vi "Strategy 4_duty cycle variation_not working.vi"() -> ()   [LabVIEW 2018]
uses:
  <vilib>/DAQmx/write.llb/DAQmx Write (Digital 1D Bool 1Chan 1Samp).vi
  <vilib>/DAQmx/create/channels.llb/DAQmx Create Channel (DO-Digital Output).vi
  <vilib>/DAQmx/miscellaneous.llb/DAQmx Fill In Error Info.vi
  <vilib>/Waveform/DWDTOps.llb/DWDT Analog to Digital.vi
  <vilib>/Waveform/DWDTOps.llb/DWDT Digital to Boolean Array.vi
  <vilib>/ptbypt/NI_PtbyPt.lvlib
  <vilib>/measure/NI_MABase.lvlib
panel:
  out "Meter":dbl(knob) scale=0.0..100.0
  out "?":bool
  in  "Boolean":bool
  in  "sample length":i32=50
  out "Waveform Chart":dbl(graph)
  in  "Set Point":dbl(slide) scale=0.0..40.0
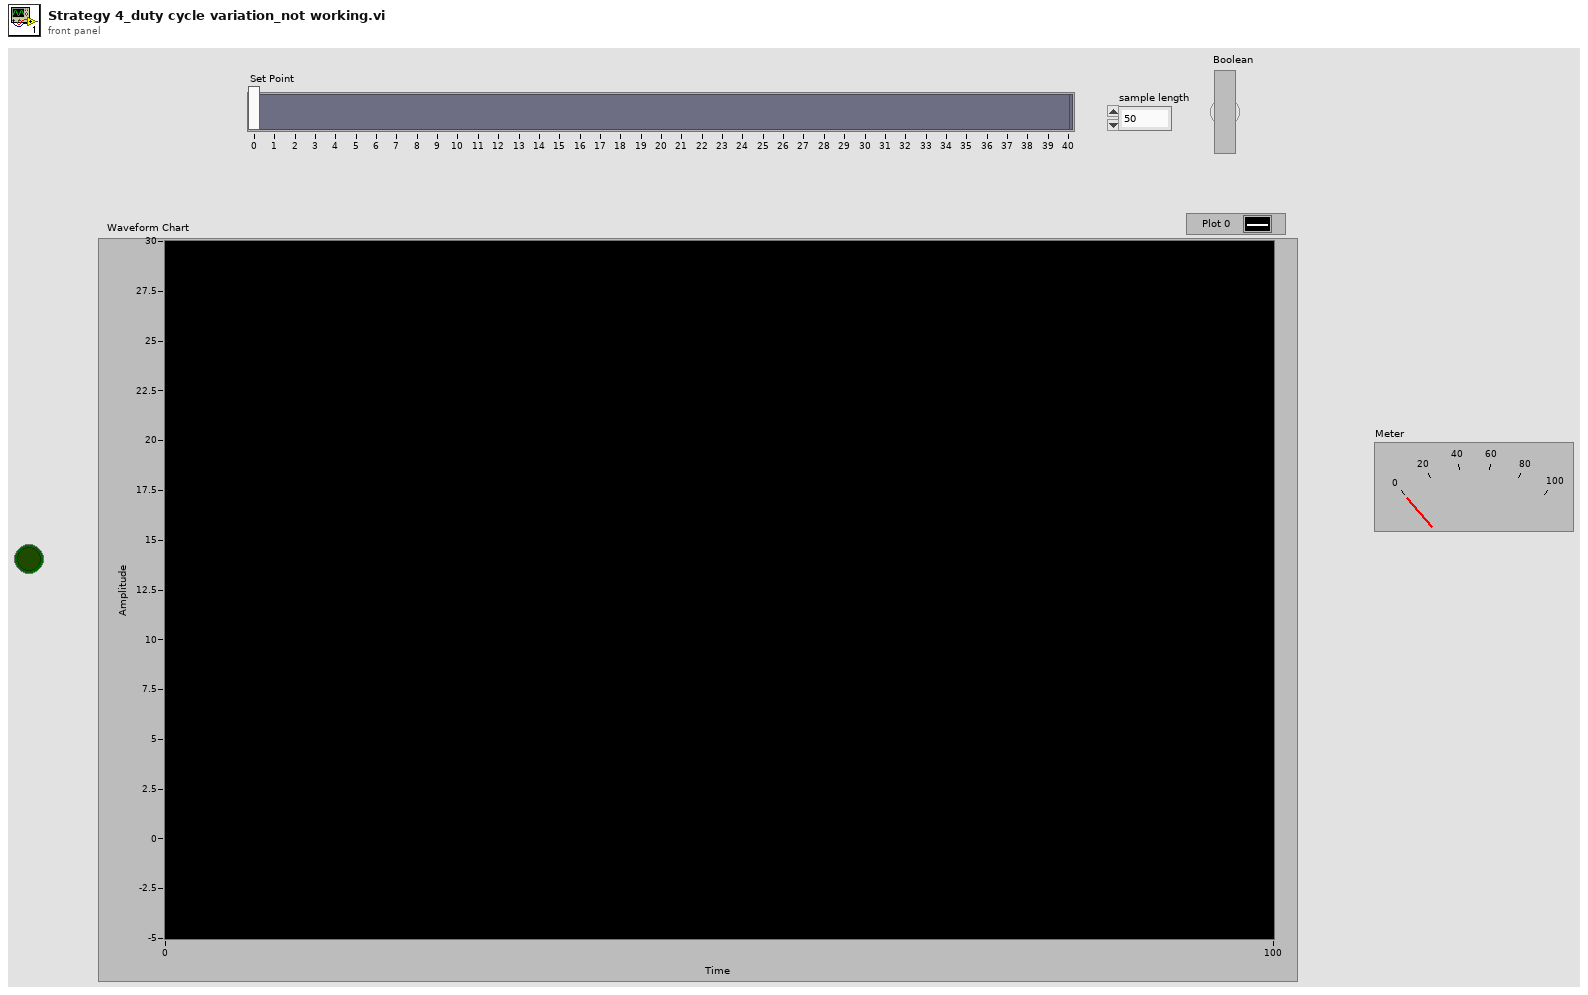
[diagram p1: front panel]
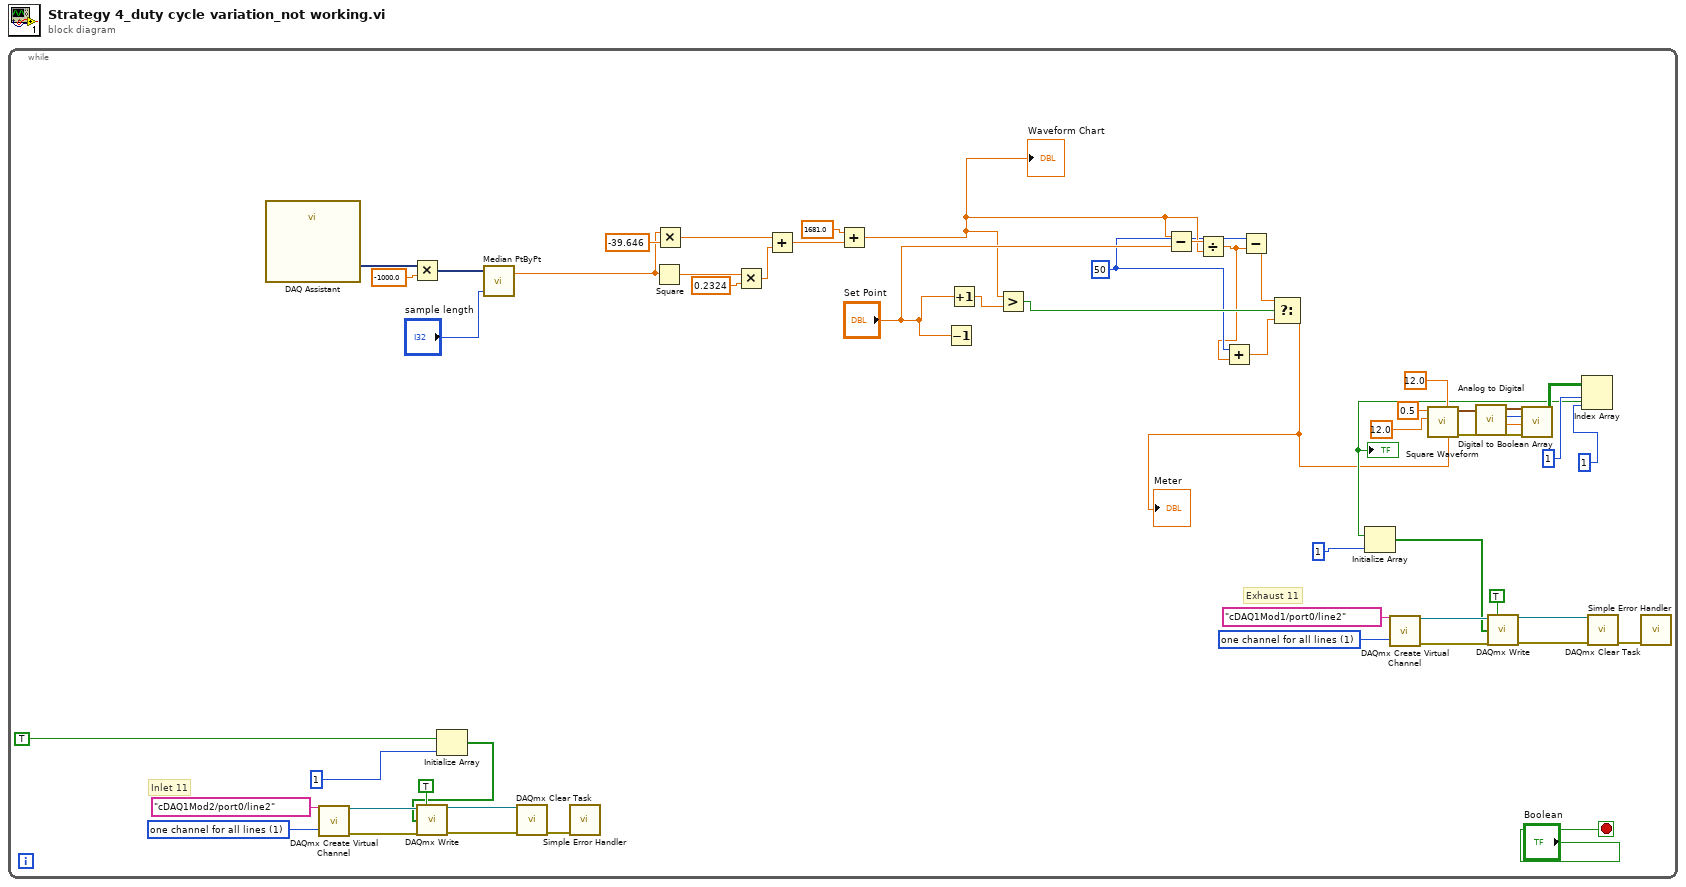
[diagram p0: block diagram]
diagram:
  n1 = while {
    stop <- "Boolean" stop-if-true
    w4 = 50
    w27 = 1 items=["one channel for each line", "one channel for all lines"] ("line grouping")
    w39 = 1 items=["one channel for each line", "one channel for all lines"] ("line grouping")
    # "Exhaust 11"
    # "Inlet 11"
    n2 = call "DAQ Assistant"() -> ("data"=w57:dynamicdata)  [unwired: 17 in, 2 out]
    n3 = call-poly <vilib>:"DAQmx Create Virtual Channel.vi"("lines"=tag "cDAQ1Mod2/port0/line2", "line grouping"=w39) -> ("task out"=w41:refnum<k21>, "error out"=w40:errorcluster)  [unwired: 12 in]
    n4 = Multiply(x=w57, y=-1000.0) -> (x*y=w48:dynamicdata)
    n5 = Initialize Array(TRUE, 1 ("dimension size")) -> (w36:bool[])
    n6 = call-poly <vilib>:"DAQmx Write.vi"("task/channels in"=w41, "auto start"=TRUE, "data"=w36, "error in"=w40) -> ("task out"=w43:refnum<k21>, "error out"=w44:errorcluster)  [unwired: 9 in, 1 out]
    n7 = call <vilib>:"Median PtByPt.vi"("sample length"="sample length", "x"=w48) -> ("median"=w47:dbl)  [unwired: 2 in, 1 out]
    n8 = call <vilib>:"DAQmx Clear Task.vi"("task in"=w43, "error in"=w44) -> ("error out"=w38:errorcluster)  [unwired: 13 in]
    n9 = call <vilib>:"Simple Error Handler.vi"("error in (no error)"=w38) -> ()  [unwired: 4 in, 5 out]
    n10 = Square(x=w47) -> (x^2=w55:dbl)
    n11 = Multiply(x=w47, y=-39.646) -> (x*y=w51:dbl)
    n12 = Multiply(x=w55, y=0.2324) -> (x*y=w52:dbl)
    n13 = Add(x=w51, y=w52) -> (x+y=w50:dbl)
    n14 = Add(x=1681.0, y=w50) -> (x+y=w7:dbl)
    "Waveform Chart" <- w7
    n15 = Decrement(x="Set Point") -> ()  [unwired: 1 out]
    n16 = Increment(x="Set Point") -> (x+1=w10:dbl)
    n17 = Greater?(x=w7, y=w10) -> (0:w5:bool)
    n18 = Subtract(x=w7, y="Set Point") -> (x-y=w8:dbl)
    n19 = Divide(x=w8, y=w7) -> (x/y=w3:dbl)
    n20 = Add(x=w4, y=w3) -> (x+y=w2:dbl)
    n21 = Subtract(x=w4, y=w3) -> (x-y=w6:dbl)
    n22 = Select(t=w6, s=w5, f=w2) -> (s? t:f=w1:dbl)
    "Meter" <- w1
    n23 = call-poly <vilib>:"DAQmx Create Virtual Channel.vi"("lines"=tag "cDAQ1Mod1/port0/line2", "line grouping"=w27) -> ("task out"=w29:refnum<k21>, "error out"=w28:errorcluster)  [unwired: 12 in]
    n24 = call <vilib>:"Square Waveform.vi"("duty cycle (%)"=w1, "offset"=12.0, "amplitude"=12.0, "frequency"=0.5) -> ("error out"=w18:errorcluster, "signal out"=w12:waveform(dbl))  [unwired: 6 in]
    n25 = call-poly <vilib>:"Analog to Digital.vi"("error in (no error)"=w18, "analog waveform"=w12) -> ("error out"=w20:errorcluster, "full-scale range (out)"=w21:dbl, "resolution (out)"=w22:i32, "digital waveform"=w19:digitalwaveform)  [unwired: 6 in]
    n26 = call-poly <vilib>:"Digital to Boolean Array.vi"("error in (no error)"=w20, "mode"=w21, "response on error"=w22, "digital waveform"=w19) -> ("boolean array"=w23:bool[][])  [unwired: 6 in, 1 out]
    n27 = Index Array(array=w23, index (row)=1, index (col)=1 ("disabled index (col)")) -> (element=w11:bool)
    "?" <- w11
    n28 = Initialize Array(w11, 1 ("dimension size")) -> (w24:bool[])
    n29 = call-poly <vilib>:"DAQmx Write.vi"("task/channels in"=w29, "auto start"=TRUE, "data"=w24, "error in"=w28) -> ("task out"=w31:refnum<k21>, "error out"=w32:errorcluster)  [unwired: 9 in, 1 out]
    n30 = call <vilib>:"DAQmx Clear Task.vi"("task in"=w31, "error in"=w32) -> ("error out"=w26:errorcluster)  [unwired: 13 in]
    n31 = call <vilib>:"Simple Error Handler.vi"("error in (no error)"=w26) -> ()  [unwired: 4 in, 5 out]
  }
